vi "DC_CNTRL_enquire_max_potential.vi"(8 "error in (no error)":errorcluster, 10 "Box Number":u16(ring), 11 "Handle":u64) -> (0 "error out":errorcluster, 2 "Max Value":dbl, 3 "Handle out":u64)   [LabVIEW 2019]
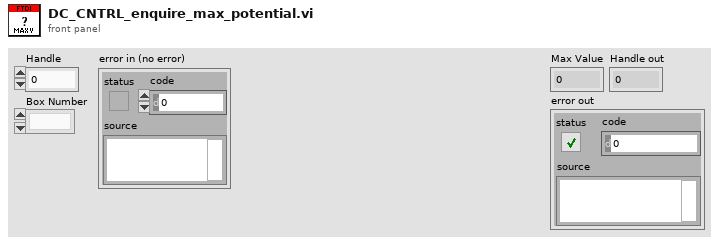
[diagram p1: front panel]
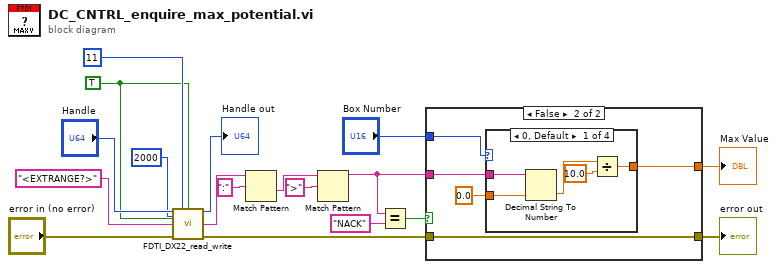
[diagram p0: block diagram]
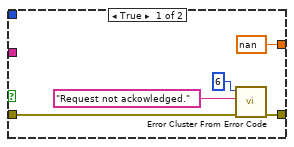
[diagram p2: hidden frame]
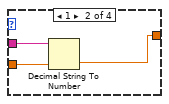
[diagram p3: hidden frame]
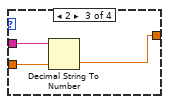
[diagram p4: hidden frame]
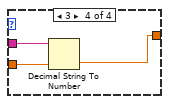
[diagram p5: hidden frame]
diagram:
  w1 = TRUE ("Read Answer?")
  n1 = call "FDTI_DX22_read_write.vi"("Handle"="Handle", "Bytes to wait for"=11, "Read Answer?"=w1, "Bytes wait timeout / ms"=2000, "Clear  RxTx Buffer?"=w1, "Write string"="<EXTRANGE?>", "error in (no error)"="error in (no error)") -> ("Handle out"=→"Handle out":u64, "Read Data"=w14:string, "error out"=w7:errorcluster)  [unwired: 6 in]
  n2 = Match Pattern(string=w14, regular expression=":") -> (after substring=w12:string)  [unwired: 1 in, 3 out]
  n3 = Match Pattern(string=w12, regular expression=">") -> (before substring=w8:string)  [unwired: 1 in, 3 out]
  n4 = Equal?(x=w8, y="NACK") -> (x = y?=w9:bool)
  n5 = case shown="False" w9 {
    tunnel: w8 -> [_ w26]
    tunnel: w7 -> [w21 w27]
    tunnel: [w20 w27] -> w3
    tunnel: "Box Number" -> [_ w25]
    tunnel: [nan w24] -> w5
    frame True {
      n6 = call <vilib>:"Error Cluster From Error Code.vi"("error in (no error)"=w21, "error message (\"\")"="Request not ackowledged." ("error message (\"\")"), "error code (0)"=6) -> ("error out"=w20:errorcluster)  [unwired: 6 in]
    }
    frame False {
      n7 = case shown="0, Default" w25 {
        tunnel: w26 -> [w33 w36 w39 w42]
        tunnel: [w30 w35 w38 w41] -> w24
        tunnel: 0.0 -> [w29 w34 w37 w40]
        frame 0, Default {
          n8 = Decimal String To Number(string=w33, default (0L)=w29) -> (number=w32:dbl)  [unwired: 1 in, 1 out]
          n9 = Divide(x=w32, y=10.0) -> (x/y=w30:dbl)
        }
        frame 1 {
          n10 = Decimal String To Number(string=w36, default (0L)=w34) -> (number=w35:dbl)  [unwired: 1 in, 1 out]
        }
        frame 2 {
          n11 = Decimal String To Number(string=w39, default (0L)=w37) -> (number=w38:dbl)  [unwired: 1 in, 1 out]
        }
        frame 3 {
          n12 = Decimal String To Number(string=w42, default (0L)=w40) -> (number=w41:dbl)  [unwired: 1 in, 1 out]
        }
      }
    }
  }
  "Max Value" <- w5
  "error out" <- w3
